vi "SetWindowRunVITransparently.vi"(8 "error in (no error)":errorcluster, 10 "\"Run VI Transparently":bool, 11 "WindowFrame in":refnum<class "WindowFrame.lvclass">) -> (0 "error out":errorcluster, 3 "WindowFrame out":refnum<class "WindowFrame.lvclass">)   [LabVIEW 2021, in "WindowFrame.lvlib" / "WindowFrame.lvclass"]
uses:
  WindowFrame.lvclass
  Action.ctl
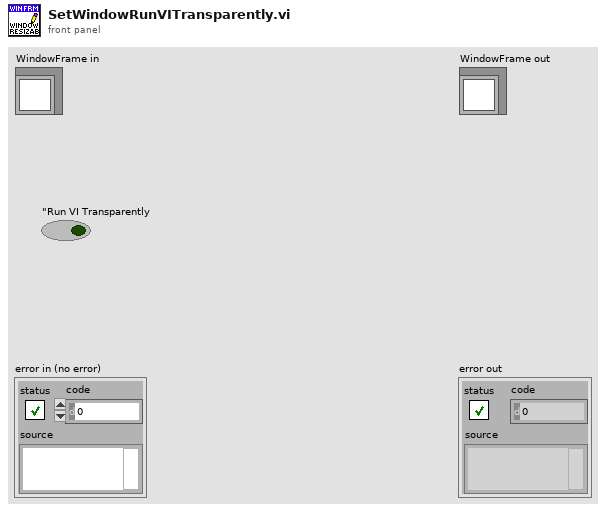
[diagram p1: front panel]
types:
  T1 = typedef "WindowFrame.lvlib/WindowFrame.lvclass/Action.ctl" = enum16{"Set Allow Runtime PopUp", "Set Behavior", "Set Closable", "Set Custom Title", "Set Highlight Return Button", "Set Is Frontmost", "Set Minimizable", "Set Minimum Size", "Set Monitor", "Set Resizable", "Set Panel Bounds", "Set Run VI Transparently", "Set Show Menu Bar", "Set State", "Set Title", "Set Title Bar Colors", "Set Title Bar Visible", "Set Transparancy", "Set Window Bounds", "Get Allow Runtime PopUp", "Get Behavior", "Get Closable", "Get Custom Title", "Get Highlight Return Button", "Get Is Frontmost", "Get Minimizable", "Get Minimum Size", "Get Monitor", "Get Panel Bounds", "Get Resizable", "Get Run VI Transparently", "Get Show Menu Bar", "Get State", "Get Title", "Get Title Bar Colors", "Get Title Bar Visible", "Get Transparancy", "Get Window Bounds", "--", "Center", "Close", "Open", "Run-Time Position:Centered", "Run-Time Position:Custom", "Run-Time Position:Get Position", "Run-Time Position:Maximized", "Run-Time Position:Minimized", "Run-Time Position:Unchanged", "---", "Insert VI", "Remove VI", "Insert VI Index", "Remove VI Index", "Exit"}
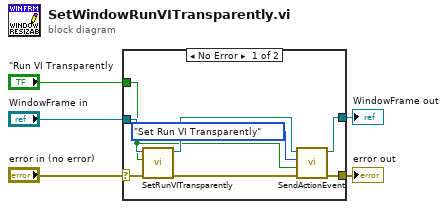
[diagram p0: block diagram]
diagram:
  n1 = case shown="No Error" "error in (no error)" {
    selector: "error in (no error)" -> [w13 w15]
    tunnel: [w11 w15] -> w4
    tunnel: [w10 w14] -> w2
    tunnel: "WindowFrame in" -> [w7 w14]
    tunnel: "\"Run VI Transparently" -> [w6 _]
    frame No Error {
      n2 = call "SetRunVITransparently.vi"("error in (no error)"=w13, "Run VI Transparently"=w6, "WindowFrame in"=w7) -> ("error out"=w12:errorcluster, "WindowFrame out"=w8:refnum<class "WindowFrame.lvclass">)  [unwired: 7 in]
      n3 = call "SendActionEvent.vi"("error in (no error)"=w12, "Variant"=w6, "Action"=Action."Set Run VI Transparently", "WindowFrame in"=w8) -> ("error out"=w11:errorcluster, "WindowFrame out"=w10:refnum<class "WindowFrame.lvclass">)  [unwired: 6 in]
    }
    frame Error {
    }
  }
  "error out" <- w4
  "WindowFrame out" <- w2
